vi "find.vi"(7 "tree (dvr) in":refnum<data-value>, 8 "error in (no error)":errorcluster, 11 "Key (search)":T2) -> (0 "error out":errorcluster, 2 "Data":T1, 3 "Found?":bool)   [LabVIEW 2015, in "binary_tree.lvlib"]
uses:
  binary_tree.lvlib
  _controls/node_key.ctl
  _controls/node_data.ctl
  _controls/tree.ctl
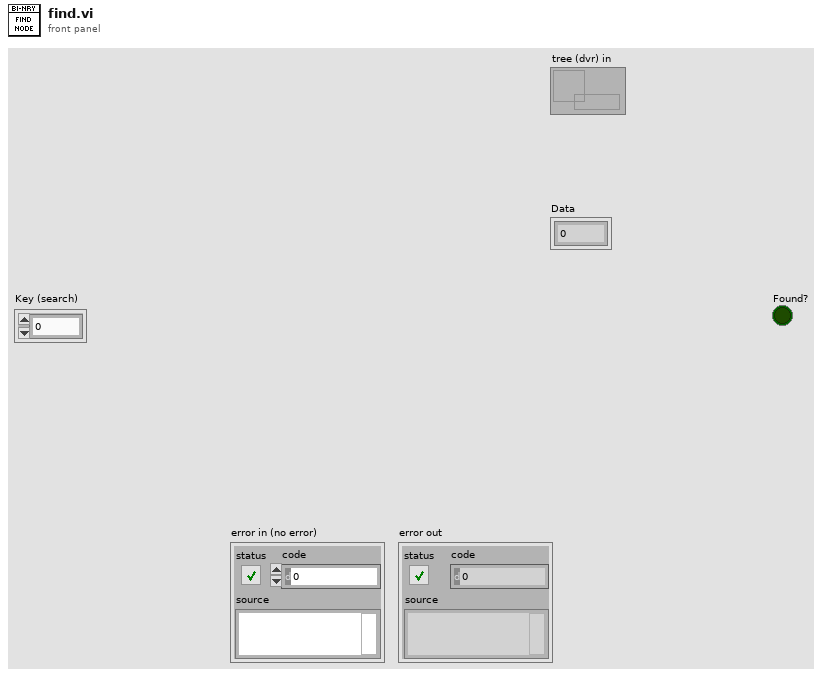
[diagram p1: front panel]
types:
  T1 = typedef "binary_tree.lvlib/node_data.ctl" = cluster{dbl}
  T2 = typedef "binary_tree.lvlib/node_key.ctl" = cluster{dbl}
  T3 = typedef "binary_tree.lvlib/tree.ctl" = cluster{"key":T2, "data":T1, "node_dvr (left)":variant, "node_dvr (right)":variant}
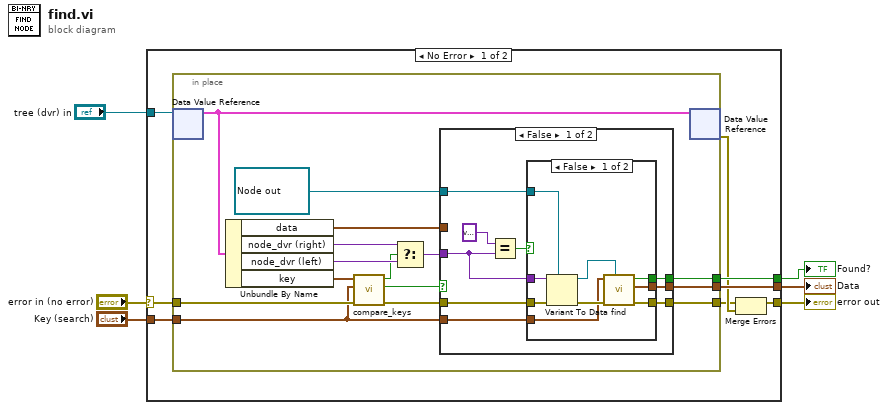
[diagram p0: block diagram]
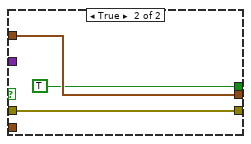
[diagram p3: hidden frame]
diagram:
  n1 = case shown="No Error" "error in (no error)" {
    selector: "error in (no error)" -> [w14 w51]
    tunnel: "Key (search)" -> [w13 _]
    tunnel: [w7 w51] -> w4
    tunnel: [w12 _] -> w3
    tunnel: [w11 _] -> w2
    tunnel: "tree (dvr) in" -> [w10 _]
    frame No Error {
      n2 = in-place {
        in-place-border: w14 -> [w24]
        in-place-border: w13 -> [w22]
        in-place-border: [w21] -> w8
        in-place-border: [w18] -> w12
        in-place-border: [w17] -> w11
        n3 = in-place-dvr #1(w10) -> (w16:T3)  [unwired: 1 out]
        n4 = Unbundle By Name(w16) -> ("data"=w19:T1, "node_dvr (right)"=w28:variant, "node_dvr (left)"=w27:variant, "key"=w26:T2)
        n5 = call "compare_keys.vi"("key (search)"=w22, "key (node)"=w26) -> ("equal"=w20:bool, "left_right"=w25:bool)  [unwired: 8 in]
        n6 = Select(t=w28, s=w25, f=w27) -> (s? t:f=w23:variant)
        n7 = case shown="False" w20 {
          tunnel: w24 -> [w37 w48]
          tunnel: w23 -> [w35 _]
          tunnel: w22 -> [w33 _]
          tunnel: [w32 w48] -> w21
          tunnel: w19 -> [_ w50]
          tunnel: [w30 w50] -> w18
          tunnel: [w31 TRUE] -> w17
          tunnel: refnum<data-value> refnum ("tree (dvr)") -> [w29 _]
          frame False {
            n8 = Equal?(x=variant ("Left"), y=w35) -> (x = y?=w34:bool)
            n9 = case shown="False" w34 {
              tunnel: w37 -> [w46 w47]
              tunnel: w35 -> [w45 _]
              tunnel: w33 -> [w39 _]
              tunnel: [w43 w47] -> w32
              tunnel: [w41 _] -> w31
              tunnel: [w42 _] -> w30
              tunnel: w29 -> [w38 _]
              frame False {
                n10 = Variant To Data(error in=w46, type=w38, Variant=w45) -> (data=w40:refnum<data-value>, error out=w44:errorcluster)
                n11 = call "find.vi"("tree (dvr) in"=w40, "error in (no error)"=w44, "Key (search)"=w39) -> ("error out"=w43:errorcluster, "Data"=w42:T1, "Found?"=w41:bool)  [unwired: 6 in]
              }
              frame True {
              }
            }
          }
          frame True {
          }
        }
        n12 = in-place-dvr #1(w16) -> (w9:errorcluster)  [unwired: 1 out]
      }
      n13 = Merge Errors(w8, w9) -> (w7:errorcluster)
    }
    frame Error {
    }
  }
  "error out" <- w4
  "Found?" <- w2
  "Data" <- w3
